vi "Add Destination.vi"(8 "error in (no error)":errorcluster, 9 "Destination type (directory)":T1, 10 "Destination label":string, 11 "SDIST in":refnum<class "NI_AB_API_DSDIST.lvclass">) -> (0 "error out":errorcluster, 3 "SDIST out":refnum<class "NI_AB_API_DSDIST.lvclass">)   [LabVIEW 2020, in "NI_AB_API_DSDIST.lvclass"]
uses:
  <vilib>/AppBuilder/AB_API/DSDIST/NI_AB_API_DSDIST.lvclass
  <vilib>/AppBuilder/AB_API/common/AB_API Destination Type.ctl
  <vilib>/AppBuilder/AB_API/SDIST/NI_AB_API_SDIST.lvclass
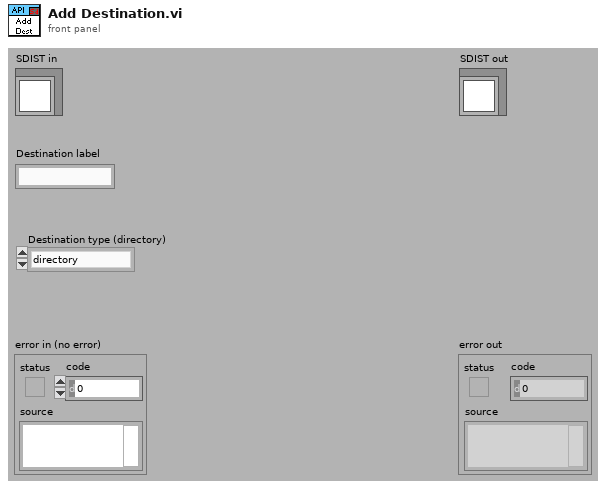
[diagram p1: front panel]
types:
  T1 = typedef "AB_API Destination Type.ctl" = enum16{"directory", "directory (preserve hierarchy)", "LLB"}
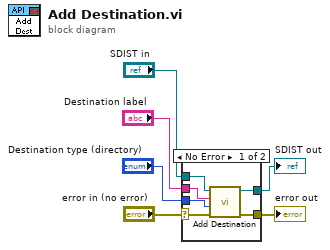
[diagram p0: block diagram]
diagram:
  n1 = case shown="No Error" "error in (no error)" {
    selector: "error in (no error)" -> [w9 w14]
    tunnel: [w10 w14] -> w5
    tunnel: [w11 w13] -> w3
    tunnel: "SDIST in" -> [w12 w13]
    tunnel: "Destination label" -> [w7 _]
    tunnel: "Destination type (directory)" -> [w8 _]
    frame No Error {
      n2 = call-parent "Add Destination.vi"("error in (no error)"=w9, "Destination type (directory)"=w8, "Destination label"=w7, "SDIST in"=w12) -> ("error out"=w10:errorcluster, "SDIST out"=w11:refnum<class "NI_AB_API_DSDIST.lvclass">)  [unwired: 6 in]
    }
    frame Error {
    }
  }
  "error out" <- w5
  "SDIST out" <- w3
